vi "Write Config File Ref.vi"(8 "error in (no error)":errorcluster, 10 "refnum in":T1, 11 "Configuration File In":refnum<class "Configuration File.lvclass">) -> (0 "error out":errorcluster, 3 "Configuration File Out":refnum<class "Configuration File.lvclass">)   [LabVIEW 2020, in "Configuration File.lvclass"]
doc: "For the configuration file interface to work, the class implementing the interface needs to save the reference to the file in the class attributes. This is an accessor for that attribute which must be implemented by the class."
uses:
  Configuration File.lvclass
  <vilib>/Utility/config.llb/Config Data RefNum.ctl
  <vilib>/Utility/config.llb/NI_LVConfig.lvlib
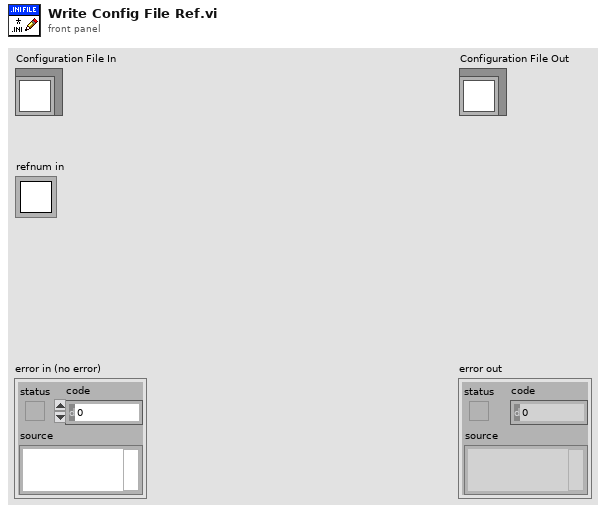
[diagram p1: front panel]
types:
  T1 = typedef "NI_LVConfig.lvlib/Config Data RefNum.ctl" = refnum<k1>
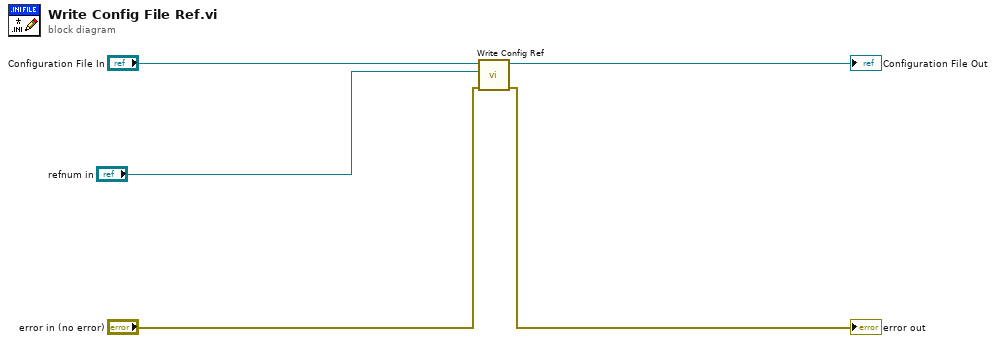
[diagram p0: block diagram]
diagram:
  n1 = call-dynamic "Write Config Ref.vi"("error in (no error)"="error in (no error)", "Reference"="refnum in", "Configuration File In"="Configuration File In") -> ("error out"=→"error out":errorcluster, "Configuration File Out"=→"Configuration File Out":refnum<class "Configuration File.lvclass">)  [unwired: 7 in]
